vi "ni579x Validate RF Filter.vi"(0 "Register Bus":refnum<class "ni579x Register Bus v1 Host.lvclass">=refnum, 1 "scope":string, 5 "frequency [Hz]":dbl format="%#_6p", 11 "Error In":errorcluster) -> (4 "Register Bus (out)":refnum<class "ni579x Register Bus v1 Host.lvclass">, 6 "coerced frequency [Hz]":dbl format="%#_6p", 15 "Error Out":errorcluster)   [LabVIEW 2015]
uses:
  <instrlib>/ni579x/Register Bus/v1/Host/ni579x Register Bus v1 Host.lvclass
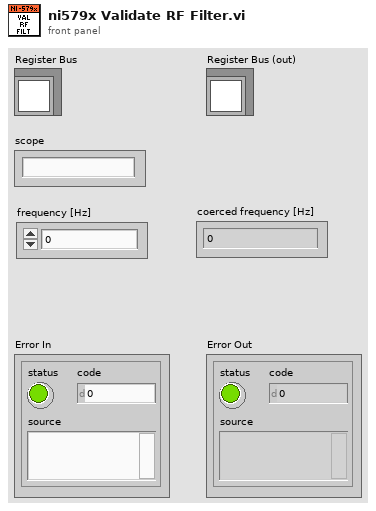
[diagram p1: front panel]
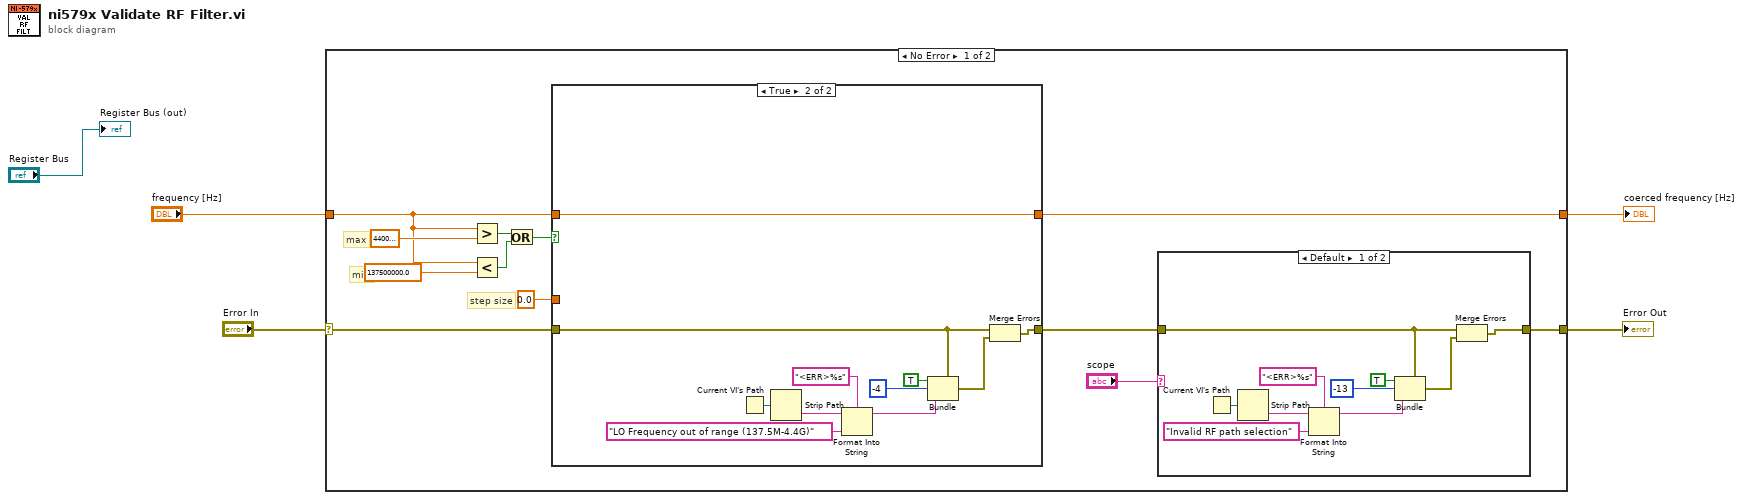
[diagram p0: block diagram]
diagram:
  n1 = case shown="No Error" "Error In" {
    selector: "Error In" -> [w10 w43]
    tunnel: [w6 w43] -> w4
    tunnel: "frequency [Hz]" -> [w12 w42]
    tunnel: [w9 w42] -> w1
    frame No Error {
      # "min"
      # "max"
      # "step size"
      n2 = Greater?(x=w12, y=4400000000.0) -> (0:w15:bool)
      n3 = Less?(x=w12, y=137500000.0) -> (x < y?=w14:bool)
      n4 = Or(x=w15, y=w14) -> (x .or. y?=w13:bool)
      n5 = case shown="True" w13 {
        tunnel: w12 -> [w29 w34]
        tunnel: 0.0 -> [_ _]
        tunnel: [w29 w34] -> w9
        tunnel: w10 -> [w30 w37]
        tunnel: [w30 w35] -> w7
        frame False {
        }
        frame True {
          n6 = Current VI's Path() -> (path=w40:path)
          n7 = Strip Path(path=w40) -> (name=w39:string)  [unwired: 1 out]
          n8 = Format Into String(format string="<ERR>%s", initial string=w39, "LO Frequency out of range (137.5M-4.4G)" ("input 1")) -> (resulting string=w38:string)  [unwired: 1 in, 1 out]
          n9 = Bundle(cluster=w37, "status"=TRUE, "code"=-4, "source"=w38) -> (w36:errorcluster)
          n10 = Merge Errors(w37, w36) -> (w35:errorcluster)
        }
      }
      n11 = case shown="Default" "scope" {
        tunnel: w7 -> [w20 w28]
        tunnel: [w18 w28] -> w6
        frame Default {
          n12 = Current VI's Path() -> (path=w22:path)
          n13 = Strip Path(path=w22) -> (name=w23:string)  [unwired: 1 out]
          n14 = Format Into String(format string="<ERR>%s", initial string=w23, "Invalid RF path selection" ("input 1")) -> (resulting string=w24:string)  [unwired: 1 in, 1 out]
          n15 = Bundle(cluster=w20, "status"=TRUE, "code"=-13, "source"=w24) -> (w19:errorcluster)
          n16 = Merge Errors(w20, w19) -> (w18:errorcluster)
        }
        frame "rx", "tx" {
        }
      }
    }
    frame Error {
    }
  }
  "Error Out" <- w4
  "coerced frequency [Hz]" <- w1
  "Register Bus (out)" <- "Register Bus"
